vi "AlliGator Square Gated IRF Characteristics Map.vi"(8 "error in (no error)":errorcluster, 11 "AlliGator Internal Variables DVR":refnum<data-value>) -> (0 "error out":errorcluster, 1 "Message":string, 3 "AlliGator Internal Variables DVR":refnum<data-value>)   [LabVIEW 2021, in "AlliGator Scripts.lvlib"]
doc: "Performs a crude square gate analysis of all ROI decays and saves the gate parameters in an ASCII file."
uses:
  AlliGator Scripts.lvlib
  Internal Variables/AlliGator Internal Variables v2.ctl
  <vilib>/vision/Image Controls.llb/IMAQ Image.ctl
  Internal Variables/AlliGator Gate Image Set.ctl
  Files/AlliGator FLI Dataset Type.ctl
  Files/AlliGator Data Series Type.ctl
  Dual-Channel Datasets/AlliGator Dataset Channel.ctl
  Settings/AlliGator Gate Arithmetic.ctl
  Source Image/AlliGator Displayed Image.ctl
  Image/Named ROI Description.ctl
  Phasor Graph/AlliGator Decay Metadata v3.ctl
  Decay Analysis/Decay Preprocessing/AlliGator Decay Background Subtraction Info.ctl
  Decay Analysis/Decay Preprocessing/AlliGator Baseline Subtraction Method.ctl
  Graphs/XY Graph/XY Graph Plot Shift Parameters.ctl
  Graphs/XY Graph/XY Graph Plot Shift Method.ctl
  Decay Analysis/Decay Preprocessing/AlliGator Decay Extrapolation Parameters.ctl
  Phasor/Calibration Phasor (m, phi).ctl
  Phasor/Phasor Reference Series.ctl
  Phasor/Phasor Calibration Map v2.ctl
  Phasor/Phasor (g, s).ctl
  Phasor Graph/AlliGator Raw Phasor Plot Data v5.ctl
  Phasor/Phasor Standard Deviation Options.ctl
  Phasor Plot/AlliGator Phasor Multi-Harmonic Data.ctl
  Phasor/Phasor Harmonic Data.ctl
  Decay Fit Parameter Map/AlliGator Decay Fit Options & Parameters v4.ctl
  Fits/IRF(X)PSED/Decay Fit Options v4.ctl
  Fits/Decay Convolution/Decay Model.ctl
  Fits/Residual Type.ctl
  Fits/IRF(X)PSED/Fit Weights Type v2.ctl
  Fits/Non-linear Fitting Method v2.ctl
  Fits/Fit Calculation Method.ctl
  Fits/Non-linear Fitting Algorithm.ctl
  Decay Analysis/Decay Fit/AlliGator Decay Fit Parameter Constraints 2.ctl
  Fits/IRF(X)PSED/Decay Fit Parameters In List.ctl
  Fits/IRF(X)PSED/MLE Baseline Offset Type.ctl
  Decay Analysis/Decay Preprocessing/AlliGator Decay Preprocessing Parameters.ctl
  Fits/IRF(X)PSED/Decay Fit Parameters & Derived Quantities List v2.ctl
  Fits/IRF(X)PSED/Decay Fit Result Constraint.ctl
  Decay Fit Parameter Map/AlliGator Parameter Maps Data.ctl
  Globals, Variables, Constants/AlliGator Variables List.ctl
  Settings/AlliGator Settings List.ctl
  Fits/Square Pulse/Square Pulse Options.ctl
  Fits/Square Pulse/Square Pulse Levels Type.ctl
  Variant/Variant to Data/Variant to U16.vi
  Globals, Variables, Constants/AlliGator Abort.vi
  <vilib>/Utility/file.llb/Write Delimited Spreadsheet (string).vi
  <vilib>/Utility/error.llb/Error Cluster From Error Code.vi
  <vilib>/ErrorRing/Error Ring.xnode
  Globals, Variables, Constants/AlliGator Globals, Variables & Constants.lvlib
  Image/Image.lvlib
  Decay Analysis/Decay Processing/AlliGator Decay Processing.lvlib
  Source Image/AlliGator Source Image.lvlib
  Strings/Strings.lvlib
  Time/Time.lvlib
  Decay Analysis/Decay Preprocessing/AlliGator Decay Preprocessing.lvlib
  Settings/AlliGator Settings.lvlib
  Fits/Fits.lvlib
  GUI/GUI.lvlib
  Utilities/Utilities.lvlib
  Variant/Variant to Data/Variant to Data.lvlib
  Phasor/Phasor.lvlib
  Files/AlliGator Files.lvlib
  Internal Variables/AlliGator Internal Variables.lvlib
  Phasor Graph/AlliGator Phasor Graph.lvlib
  Graphs/XY Graph/XY Graph Add-Ons.lvlib
  Phasor Plot/AlliGator Phasor Plot.lvlib
  Decay Analysis/Decay Fit/AlliGator Decay Fit.lvlib
  Dual-Channel Datasets/AlliGator Dual-Channel Datasets.lvlib
  Decay Fit Parameter Map/AlliGator Decay Fit Parameter Map.lvlib
panel:
  # "see the AlliGator License on the block diagram (Ctrl+E or Window:Show Block Diagram)"
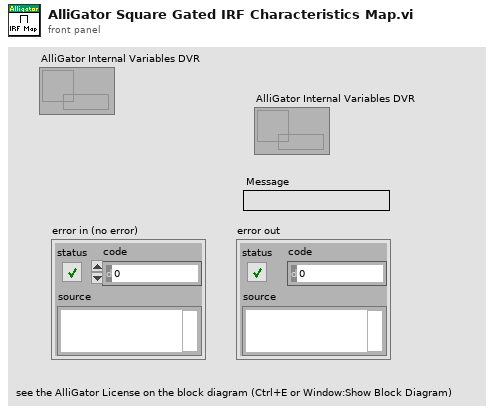
[diagram p1: front panel]
types:
  T1 = typedef "AlliGator Globals, Variables & Constants.lvlib/AlliGator Variables List.ctl" = enum16{"---- GUI ----", "GUI:Initialization Status", "GUI:State Indicators Refnum", "GUI:Original AlliGator Menu Items", "GUI:Current Action Loop State", "GUI:Script in progress", "GUI:Playback", "GUI:Loop Playback", "GUI:Search ROI Used", "GUI:Search ROI", "Decay Graph Max Legend Size", "Intensity Graph Max Legend Size", "Decay Statistics Graph Max Legend Size", "Phasor Graph Max Legend Size", "Phasor Ratio Graph Max Legend Size", "Lifetime Graph Max Legend Size", "---- Files ----", "Files:Export Dataset Frames as Individual Files", "Files:Show Batch Export Help Balloons", "Files:Frames in Dataset", "Files:ptu File Frame Start Indices", "Files:Current Frame in Dataset", "Files:Current Frame Timestamp", "Files:Dataset Loaded", "Files:Dataset Metadata", "Files:Dataset Channel", "Files:Dataset Data Description", "Files:Background Dataset Metadata", "Files:Background Dataset Channel", "Files:Background Dataset Data Description", "Files:Background File Subtraction", "Files:Background File Path", "Files:Background File Pile-up Correction", "Files:Background File Pixel Well Capacity", "Files:Background File Scaling Factor", "Files:Current Dataset Load Settings", "Files:Dataset Path", "Files:ICCD-specific Information", "Files:Macrotime Gate Separation", "------ Python Plugins ------", "Python Plugins:Information", "Python Plugins:Python Session", "Python Plugins:Valid Python Session?", "---- Source Image ----", "Source Image:ROIs", "Source Image:Current ROI", "Source Image:ROI Event Refnum", "X_Source Image:Display Range", "X_Source Image:Palette Information", "X_Source Image:Type of Displayed Image", "X_Time Gate Slider", "Source Image:Palette List", "Source Image:Scale", "Source Image:ROI Overlay Color", "Source Image:Overlay to Erase", "Source Image:Is Displayed Image Accumulated", "Source Image:White Light Image Modified", "Source Image:Mask Image Modified", "---- Image Profile Window ----", "Image Profile:Window Event Refnum", "Image Profile:IntensityType", "Image Profile:Intensity Average Type", "Image Profile:Intensity-weighted SDV", "Image Profile:Box Profile Type", "Image Profile:Window Open", "Image Profile:Plotted Fit Parameter", "------ Phasor Graph -------", "Phasor Graph:Show Line", "---- Phasor Plot ---", "Phasor Plot:Parameters Changed", "Phasor Plot:FLI Dataset Modified since last Calculation", "Phasor Harmonics Data", "Selected Phasor Harmonics", "Phasor Harmonic Manager Event Refnum", "Phasor Plot:ROIs", "Phasor Plot:Current ROI", "Phasor Plot:ROI Event Refnum", "Phasor Plot:Image Reference Points", "Phasor Plot:Computed", "Phasor Plot:Palette Information", "Phasor Plot:Palette List", "Phasor Plot:Phasor Ratio Palette Information", "Phasor Plot:Phasor Ratio Palette List", "Phasor Plot:Image Scale", "Phasor Plot:Image Overlay to Erase", "Phasor Plot:Image Elements to Update", "Phasor Plot:Current Calculation Parameters", "Phasor Plot:Current Calibration Options", "Phasor Plot:Reset Cumulated Phasor Plot", "Phasor Plot:Reference 1", "Phasor Plot:Lifetime Reference 1", "Phasor Plot:Reference 1 Frequency", "Phasor Plot:Reference 2", "Phasor Plot:Lifetime Reference 2", "Phasor Plot:Reference 2 Frequency", "---- Decay Analysis ----", "Number of Selected Decays to Fit", "LS Fit Results", "LAR Fit Results", "BS Fit Results", "Last Decay Max - Min", "Best Fit Parameters", "Best Fit Parameter Names", "Actual Size X", "Actual Size Y", "Binning X", "Binning Y", "Actual # Gates", "Dataset Number", "Gates to...", "Gates Skipped", "Gates to keep", "Gate Step", "Gate Separation", "Reversed Gates", "Pile-up Correction", "Pixel Well Capacity", "Background Subtracted", "Background Subtraction Method", "Background Definition Range", "Background File (deprecated)", "Number of Dataset Accumulated", "Array of Accumulated Dataset Paths", "Do Averaged Datasets", "Destination File Path", "Process Plot Target", "Use 1/D as Phasor Frequency", "---- Decay Fit Parameter Map -----", "Decay Fit Parameter Map:Palette Information", "Decay Fit Parameter Map:Palette List", "Decay Fit Parameter Map:X Resolution", "Decay Fit Parameter Map:Y Resolution", "Decay Fit Parameter Map:Use Decay Fit Result Constraints", "Decay Fit Parameter Map:Decay Fit Result Constraints", "Decay Fit Parameter Map:Decay Fit Result Constraints Applied", "---- Parameter Map ----", "Parameter Map:Palette Information", "Parameter Map:Palette List", "------- Local Decay Window ---------", "Local Decay Graph Window:Event Refnum", "Local Decay Graph Window:Use normalized IRF for convolution", "----- Miscellaneous ----", "Misc:Skippable Dialog Windows Status"}
  T2 = typedef "IMAQ Image.ctl" = refnum<image>
  T3 = typedef "AlliGator Settings.lvlib/AlliGator Settings List.ctl" = enum16{"GUI:Visible Settings Tab", "GUI:Last Run Version", "Source Image:Use Image Histogram for Contrast", "Source Image:Low Count Pixels Rejection Options", "Source Image:High Count Pixels Rejection Options", "Source Image:Use Image Brightness", "Source Image:Blend Overlay with Image Background", "Source Image:Use Fixed ROI Diameter", "Source Image:ROI Diameter", "Source Image:ROI Center Color", "Source Image:Peak Threshold", "Source Image:Intensity Threshold", "Source Image:Image Binning Options", "Source Image:Image Smoothing Options", "Source Image:Image Histogram Active", "Source Image:Invert Binary Mask", "Source Image:Hot Pixel Removal", "Source Image:Overlay Analyzed ROI Center", "Source Image:Auto-Adjust Contrast", "Source Image:Histogram Lower Percentile", "Source Image:Histogram Upper Percentile", "Source Image:Save Source Image", "Source Image:Scale Bar Options", "Source Image:Image Resolution (Pixel Size)", "Source Image:Flatfield Correction", "Source Image:Show Dead Left Columns Correction", "Source Image:Dead Left Columns Correction", "Source Image:Image Pre-Processing Operations Order", "Source Image:Overlay ROI Median", "Source Image:Median Overlay Color", "Data Information:Gate Width", "Data Information:Nanotime Gate Separation", "Data Information:Macrotime Gate Separation", "Data Information:Gate Step", "Data Information:# Gates", "Data Information:Gate Image Exposure", "Data Information:Gate Image Integration", "Data Information:Gates to Skip", "Data Information:Gates to Keep", "Data Information:Define Gates to", "Data Information:Channel Name", "Data Information:Available Channel Names", "Data Information:Channel Arithmetic", "Data Information:Background File Subtraction", "Data Information:Background File", "Data Information:Background Scaling Factor", "Data Information:Background Pile-up Correction", "Data Information:Background Pixel Well Capacity", "Data Information:Laser Period", "Data Information:SYNC Period", "Data Information:Pile-up Correction", "Data Information:Pixel Well Capacity", "Data Information:Dataset Scaling Factor", "Fluorescence Decay_Decay Pre-Processing:Reverse Gates", "Fluorescence Decay_Decay Pre-Processing:Verbose Decay Pre-Processing", "Fluorescence Decay_Decay Pre-Processing:Use Decay Pre-Processing", "Fluorescence Decay_Decay Pre-Processing:Background Subtraction", "Fluorescence Decay_Decay Pre-Processing:Background Definition Range", "Fluorescence Decay_Decay Pre-Processing:Baseline Subtraction Method", "Fluorescence Decay_Decay Pre-Processing:Decay Pre-Processing Operations Order", "Fluorescence Decay_Decay Pre-Processing:Smoothing Parameter", "Fluorescence Decay_Decay Pre-Processing:Shift Decay", "Fluorescence Decay_Decay Pre-Processing:Decay Shift Parameters", "Fluorescence Decay_Decay Pre-Processing:Fold Decay", "Fluorescence Decay_Decay Pre-Processing:# Folds", "Fluorescence Decay_Decay Pre-Processing:1-Normalize Decay", "Fluorescence Decay_Decay Pre-Processing:[0-1]-Normalize Decay", "Fluorescence Decay_Decay Pre-Processing:Smoothen Decay", "Fluorescence Decay_Decay Pre-Processing:Extrapolate Decay", "Fluorescence Decay_Decay Pre-Processing:Use Periodicity", "Fluorescence Decay_Decay Pre-Processing:Use Cursors", "Fluorescence Decay_Decay Pre-Processing:Tail Fraction", "Fluorescence Decay_Decay Pre-Processing:Head Fraction", "Fluorescence Decay_Decay Pre-Processing:Additional Points", "Fluorescence Decay_Decay Pre-Processing:Straighten Decay", "Fluorescence Decay_Decay Pre-Processing:Constant Background", "Fluorescence Decay_Decay Pre-Processing:Pixel-Normalize Decay", "Fluorescence Decay_Advanced Analysis:Extract IRF instead of Decay", "Fluorescence Decay_Advanced Analysis:IRF Extraction Options", "Fluorescence Decay_Advanced Analysis:IRF Optimization Options", "Fluorescence Decay_Advanced Analysis:Square Pulse Options", "Fluorescence Decay_Advanced Analysis:IRF Order", "Fluorescence Decay_Advanced Analysis:IRF Time Constants", "Fluorescence Decay_Advanced Analysis:Wavelet Analysis Options", "Fluorescence Decay_Advanced Analysis:Average Lifetime Options", "Fluorescence Decay_Fit Options:Fit Options", "Fluorescence Decay_Fit Options:Use Legacy Fitting Approach", "Fluorescence Decay_Fit Options:Use Data Information Laser Period", "Fluorescence Decay_Fit Parameters:Displayed Fit Parameters", "Fluorescence Decay_Fit Parameters:Fit Parameter Constraints", "Fluorescence Decay_Fit Parameters:Export Tabulated Results", "Fluorescence Decay_Fit Parameters:MLE Baseline Offset Type", "Fluorescence Decay_Fit Parameters:MLE Baseline Offset", "Fluorescence Decay_Fit Parameters:Guess Parameter Names", "Fluorescence Decay_Fit Parameters:Guess Parameter Values", "Fluorescence Decay_Fit Parameters:Guess Parameters Options", "Fluorescence Decay_Fit Parameters:Optimal Offset Selection Criterion", "Fluorescence Decay_Styles:Show Last Decay Only", "Fluorescence Decay_Styles:Decay Graph Color Array", "Fluorescence Decay:Decay Graph Active", "Fluorescence Decay Statistics:Min Peak Value", "Fluorescence Decay Statistics:Reject Low Decay Peak Pixels", "Fluorescence Decay Statistics:Reject High Decay Peak Pixels", "Fluorescence Decay Statistics:Max Peak Value", "Time Traces:Use File Timestamp", "Time Traces:Time Step", "Time Traces:Use Intensity Correction File", "Time Traces:Intensity Correction File", "Phasor Plot:Phasor Plot Smoothing Options", "Phasor Plot:Phasor Plot Size", "Phasor Plot:Phasor Plot Graphics Options", "Phasor Plot:Cumulative Phasor Plot", "Phasor Plot:Use Phasor Brightness", "Phasor Plot:Blend Overlay with Phasor Background", "Phasor Plot:Save Phasor Plot", "Phasor Plot:Show References", "Phasor Plot:Phasor Ratio Decay Range", "Phasor Plot:Exponential Fading", "Phasor Plot:Phasor Ratio Reference Colors", "Phasor Plot:Reference Radius", "Phasor Plot:Show Color Map Vertices", "Phasor Plot:Phasor Plot Active", "Phasor Plot:Phasor Ratio Color Map Type", "Phasor Plot:Phasor Ratio Color Map", "Phasor Plot:Phasor Ratio Display Range", "Phasor Plot:Selected Image ROI(s)", "Phasor Plot:All Image ROIs", "Phasor Plot:Selected Phasor Plot ROI(s)", "Phasor Plot:All Phasor Plot ROIs", "Phasor Plot:Phasor Ratio Color-Coded Quantity", "Phasor Plot:Store Phasor Harmonics", "Phasor Plot:Draw Reference Segment", "Phasor Plot:User-Defined Quantity", "Phasor Plot:Color Scale High Color", "Phasor Plot:Color Scale Low Color", "Phasor Plot:Intensity-weighted Phasor Plot", "Phasor Graph:Phasor Frequency", "Phasor Graph:Phasor Ratio Type", "Phasor Graph:Pixel-level Phasor Computation", "Phasor Graph:Save Phasor Graph", "Phasor Graph:Phasor Graph Active", "Phasor Graph:Phasor SDV Options", "Phasor Graph:Intensity-weighted Phasor Graph", "Phasor Graph:Define Shortest Lifetime as", "Phasor Calibration:Use Backup Calibration if needed", "Phasor Calibration:Backup Calibration Type", "Phasor Calibration:Calibration Type", "Phasor Calibration:Calibration Lifetime", "Phasor Calibration:Calibration Map Algorithm", "Single-Exponential Phasor Locus (SEPL):Gate Parameters", "Single-Exponential Phasor Locus (SEPL):User-defined Gate", "Single-Exponential Phasor Locus (SEPL):User-defined IRF", "Single-Exponential Phasor Locus (SEPL):Phasor Parameters", "Single-Exponential Phasor Locus (SEPL):Decay & IRF Parameters", "Single-Exponential Phasor Locus (SEPL):Display Parameters", "Lifetime Analysis:Decay Analysis Parameters", "Lifetime Analysis:Lifetime Map Active", "Plugins:Python Settings", "Miscellaneous:Verbose Mode", "Miscellaneous:Beep after Script", "Miscellaneous:Saved Image File Format", "Miscellaneous:Exported Gate Image Settings", "Miscellaneous:Include Loading in Timing", "Miscellaneous:Verbose Settings Mode", "Miscellaneous:Histogram Options", "Miscellaneous:Beep on Error", "Miscellaneous:# Logical Processors Used", "Miscellaneous:ROI Description Max Characters", "Miscellaneous:Verbose Error Mode", "Miscellaneous:Transparent Mask Color"}
  T4 = typedef "Fits.lvlib/Square Pulse Options.ctl" = cluster{"Method":T5, "# Bins":i32, "Threshold %":dbl, "Center on Midpoint":bool, "Smoothen Plot":bool}
  T5 = typedef "Fits.lvlib/Square Pulse Levels Type.ctl" = enum16{"Mode", "Mean"}
  T6 = typedef "Image.lvlib/Named ROI Description.ctl" = cluster{"ROI Descriptor":T7, "ROI Name":string, "Overlay Color":u32}
  T7 = typedef "ROI Descriptor" = cluster{"Global Rectangle":i32[], "Contours":cluster{"ID":enum32{"External", "Internal"}, "Type":u32, "Coordinates":i32[]}[]}
  T8 = typedef "AlliGator Internal Variables.lvlib/AlliGator Internal Variables v2.ctl" = cluster{"----------------------------- Images -----------------------------":u8, "Displayed Image":T2, "White Light Image":T2, "Mask Image":T2, "ROI Mask Image":T2, "Current Dataset Images 1":T9, "Background Dataset Images 1":T9, "Current Dataset Images 2":T9, "Background Dataset Images 2":T9, "Current Dataset Arithmetic Images":T9, "Accumulated Dataset Images 1":T9, "Accumulated Dataset Images 2":T9, "Accumulated Dataset Arithmetic Images":T9, "----------------------------- File Paths -----------------------------":u8, "Phasor Plot Image":T2, "Decay Fit Parameter Map Image":T2, "Parameter Map Image":T2, "Single Data Point Path":path, "White Light Image Path":path, "Mask Image Path":path, "Time-Series Folder":path, "[Time-Series Paths]":path[], "----------------------------- FLI Dataset -----------------------------":u8, "Current Dataset":i32, "Single Dataset Type":T10, "Current Folder":string, "AlliGator Data Series Type":T11, "# Datasets":i32, "Dual-Channel Dataset":bool, "Selected Channel Name":string, "Dataset Channel":T12, "Channel Arithmetic":T13, "Dual-Channel Background Dataset":bool, "Background Channel":T12, "Dual-Channel Accumulated Dataset":bool, "Start Time":dbl, "[Time-Series Timestamps]":dbl[], "[Intensity Corrections]":dbl[], "Time Series Script":bool, "Type of Displayed Image":T14, "Gate Image Slide":u16, "# Gates":i32, "ROIs":T6[], "----------------------------- Decays -----------------------------":u8, "ROI Decay":cluster{"t Array":dbl[], "I Array":dbl[]}, "Valid Decay":bool, "Decay  Metadata":T15, "Reference Decay Plot Name":string, "Reference Decay":cluster{"t Array":dbl[], "I Array":dbl[]}, "Decay Shift Plot":cluster{"Time Stamps":dbl[], "Decay Shifts":dbl[]}, "[Decays Max Values]":sgl[], "[Decays Min Values]":sgl[], "----------------------------- Calibration -----------------------------":u8, "Calibration Phasor":T21, "Calibration Phasor Series":T22, "Phasor Calibration Map":T23, "Calibration Map MD5 Digest":string, "----------------------------- Phasor Graph -----------------------------":u8, "Last Raw Phasor":T24, "Last Calibrated Phasor":T24, "Last Calibrated Phasor SDV":T24, "Phasor Graph:Phasor Plot":cluster{"g Array":dbl[], "s Array":dbl[]}, "Phasor Graph:Phasor SDV Plot":cluster{"g Array":dbl[], "s Array":dbl[]}, "[Phasor Graph:Raw Phasor Plots]":T25[], "Phasor Plot locked to Ref 1":i32, "[Phasor Plot(s) locked to Ref 1]":i32[], "[Phasor Plot(s) locked to Ref 2]":i32[], "[Pixel Phasors]":T24[], "----------------------------- Phasor Plot -----------------------------":u8, "[[Sum Image]]":dbl[][], "[[CSG Phasors]]":csg[][], "[[Valid Pixel?]]":bool[][], "[[Phasor Ratios]]":dbl[][], "[[Average Lifetimes]]":dbl[][], "Amplitude Weighted Average Lifetime":bool, "I/m/phi Dataset":cluster{"I/m/phi Dataset?":bool, "Base Frequency":dbl[unit], "Harmonic Orders":u8[]}, "Multi Phasor Plot Data":T27, "----------------------------- Decay Fit Parameter Map -----------------------------":u8, "Decay Fit Options & Parameters":T29, "Fit Options: Decay Preprocessing Parameters":T40, "Fit Options: Reference Decay":cluster{"t Array":dbl[], "I Array":dbl[]}, "Is Full Image Parameters Map":bool, "Is Single-Pixels Parameters Map":bool, "NLSF Parameters Map X Resolution":i32, "NLSF Parameters Map Y Resolution":i32, "[Single Decay Fit Parameters]":dbl[], "Fit Model":T31, "[[Multiple Decays Fit Parameters]]":dbl[][], "[[Multiple Decays Fit Parameter SDVs]]":dbl[][], "[[IRFs]]":dbl[][], "[ROI Descriptors]":T7[], "IRF Array Time Axis":dbl[], "Decay Array Time Axis":dbl[], "[Decay Fit Parameter Names]":T41[], "[Decay Sum]":dbl[], "Array of Decay Fit Result Constraints":T42[], "Selected ROIs Array":bool[], "----------------------------- Parameter Maps -----------------------------":u8, "[Map Set Names]":string[], "[Parameter Maps]":T43[], "[[User-defined Quantities]]":dbl[][], "User-defined Quantity":string}
  T9 = typedef "AlliGator Internal Variables.lvlib/AlliGator Gate Image Set.ctl" = cluster{"SGL Gate Images":T2[], "SGL Sum Image":T2, "SGL Max Image":T2, "SGL Min Image":T2}
  T10 = typedef "AlliGator Files.lvlib/AlliGator FLI Dataset Type.ctl" = enum16{"HDF5 FLI Dataset", "Gate Image Folder", ".sdt FLI Dataset (Becker & Hickl)", ".ptu FLI Dataset (PicoQuant)", "SS1 FLI Dataset", "SS2 FLI Dataset", "I/m/phi Dataset", ".bin FLI Dataset (PicoQuant Binned)", ".bin FLI Dataset (Piccolo Binned)", ".mat FLI Dataset"}
  T11 = typedef "AlliGator Files.lvlib/AlliGator Data Series Type.ctl" = enum16{"Not a Supported Series", "Gate Images Folder Series", "SwissSPAD 2 Dataset Series", "B&H FLI Dataset Series", "PicoQuant PTU FLI Dataset Series", "PicoQuant BIN FLI Dataset Series", "Piccolo hist BIN FLI Dataset Series", "HDF5 FLI Dataset Series"}
  T12 = typedef "AlliGator Dual-Channel Datasets.lvlib/AlliGator Dataset Channel.ctl" = enum16{"G2", "INT"}
  T13 = typedef "AlliGator Settings.lvlib/AlliGator Gate Arithmetic.ctl" = enum16{"None", "INT-G2", "G2/INT*<INT>", "(1 - G2/INT)*<INT>"}
  T14 = typedef "AlliGator Source Image.lvlib/AlliGator Displayed Image.ctl" = enum16{"Single Gate", "Sum of All Gates", "Max of All Gates", "Min of All Gates", "-", "White Ligth Image", "Mask Image"}
  T15 = typedef "AlliGator Phasor Graph.lvlib/AlliGator Decay Metadata v3.ctl" = cluster{"ROI Descriptor":T7, "ROI Center":cluster{"X":i32, "Y":i32}, "Decay Background Subtraction Info":T16, "Decay Reverted":bool, "Decay Smoothened":bool, "Decay Straightened":bool, "Fitted Tau (Decay Straightening)":dbl, "Decay Shift Parameters":T18, "Decay Shifted":bool, "Decay Extrapolated":bool, "Decay Extrapolation Parameters":T20, "Decay Normalized":bool, "Fold Decay":bool, "# Folds":u32}
  T16 = typedef "AlliGator Decay Preprocessing.lvlib/AlliGator Decay Background Subtraction Info.ctl" = cluster{"Laser Period":dbl[unit], "Gate Duration":dbl[unit], "Baseline Subtraction Method":T17, "Background Definition Range":cluster{"Min Gate":dbl[unit], "Max Gate":dbl[unit]}, "Total Intensity w/o Bkgd Subtraction":dbl, "Bkgd-subtracted Intensity (exp)":dbl, "# Data Points":i32, "Background/Gate":dbl, "Fitted Lifetime":dbl[unit], "Bkgd-subtracted Intensity (theo)":dbl}
  T17 = typedef "AlliGator Decay Preprocessing.lvlib/AlliGator Baseline Subtraction Method.ctl" = enum16{"Mean", "Min", "Square Gated Single-Exponential", "File", "Constant"}
  T18 = typedef "XY Graph Add-Ons.lvlib/XY Graph Plot Shift Parameters.ctl" = cluster{"Type":T19, "Shift":dbl[unit], "Threshold":dbl, "Rotate":bool}
  T19 = typedef "XY Graph Add-Ons.lvlib/XY Graph Plot Shift Method.ctl" = enum16{"Default", "CFD", "Threshold", "Cross-Correlation"}
  T20 = typedef "AlliGator Decay Preprocessing.lvlib/AlliGator Decay Extrapolation Parameters.ctl" = cluster{"Additional Points":u32, "Head Fraction":dbl, "Fitted Tau":dbl, "Use Periodicity":bool, "Use Cursors":bool, "Tail Fraction":dbl}
  T21 = typedef "Phasor.lvlib/Calibration Phasor (m, phi).ctl" = cluster{"m":dbl, "phi":dbl, "Phasor Frequency":dbl[unit], "Reference Lifetime":dbl[unit]}
  T22 = typedef "Phasor.lvlib/Phasor Reference Series.ctl" = cluster{"m Array":dbl[], "phi Array":dbl[], "Phasor Frequency":dbl[unit], "Calibration Lifetime":dbl[unit]}
  T23 = typedef "Phasor.lvlib/Phasor Calibration Map v2.ctl" = cluster{"Phasor Frequency":dbl[unit], "Calibration Lifetime":dbl[unit], "ROI Centers":cluster{"X":i32, "Y":i32}[], "ROI Descriptors":T7[], "Map Resolution X":i32, "Map Resolution Y":i32, "z Array":cdb[]}
  T24 = typedef "Phasor.lvlib/Phasor (g, s).ctl" = cluster{"g":dbl, "s":dbl}
  T25 = typedef "AlliGator Phasor Graph.lvlib/AlliGator Raw Phasor Plot Data v5.ctl" = cluster{"Phasor Plot Name":string, "Raw Phasor Plot":T24[], "Phasor Frequency":dbl[unit], "[Decay Metadata]":T15[], "Raw Phasor Plot SDV":T24[], "Phasor SDV Options":T26, "[Calibration Phasor]":T21[], "Intensity Array":dbl[]}
  T26 = typedef "Phasor.lvlib/Phasor Standard Deviation Options.ctl" = cluster{"Compute Estimated SDV":bool, "# Replicas":u32, "Use Estimated Average Phasor":bool}
  T27 = typedef "AlliGator Phasor Plot.lvlib/AlliGator Phasor Multi-Harmonic Data.ctl" = cluster{"Base Frequency":dbl[unit], "# Harmonics":u8, "Harmonic Orders":u8[], "Phasor Plot Settings Checksum":u64, "Phasor Harmonic Data Array":T28[]}
  T28 = typedef "Phasor.lvlib/Phasor Harmonic Data.ctl" = cluster{"Phasor Harmonic Name":string, "Phasor Plot Settings Checksum":u64, "Phasor Frequency":dbl[unit], "Base Frequency":dbl[unit], "Harmonic Order":u8, "Phasor Plot Parameters":string, "Phasor Array [[CSG]]":csg[][], "Dataset File Path":path}
  T29 = typedef "AlliGator Decay Fit Parameter Map.lvlib/AlliGator Decay Fit Options & Parameters v4.ctl" = cluster{"SYNC Period":dbl[unit], "Fit Options":T30, "Fit Parameter Constraints":T37[], "MLE Baseline Offset":dbl, "MLE Baseline Offset Type":T39}
  T30 = typedef "Fits.lvlib/Decay Fit Options v4.ctl" = cluster{"Show Fit Residuals":bool, "Fit Model":T31, "Residual Type":T32, "Max Decay Percentile":dbl, "Min Decay Percentile":dbl, "Show Full Decay":bool, "Weights":T33, "Fitting Method":T34, "Compute Parameter Uncertainties":bool, "Periodic Boundaries":bool, "Model Calculation":T35, "Period":dbl[unit], "Termination Criteria":cluster{"Max Iterations":i32, "Max Function Calls":i32, "Max Time":dbl[unit], "Function Tolerance":dbl, "Parameter Tolerance":dbl, "Gradient Tolerance":dbl, "Min Lambda":dbl, "Max Lambda":dbl, "Initial Tick Count":u32}, "Offset Resolution":dbl[unit], "Use Local IRF":bool, "Fitting Algorithm":T36, "Show Confidence Interval ":bool, "Confidence Level":dbl}
  T31 = typedef "Fits.lvlib/Decay Model.ctl" = enum16{"1-Exponential", "2-Exponentials"}
  T32 = typedef "Fits.lvlib/Residual Type.ctl" = enum16{"Standard", "Normalized", "Reduced"}
  T33 = typedef "Fits.lvlib/Fit Weights Type v2.ctl" = enum16{"Unweighted", "1/Variance (Neyman)", "1/Variance (Pearson)", "Best of All"}
  T34 = typedef "Fits.lvlib/Non-linear Fitting Method v2.ctl" = enum16{"Least Square", "Least Absolute Residual", "Bisquare", "MLE", "-", "Best of All"}
  T35 = typedef "Fits.lvlib/Fit Calculation Method.ctl" = enum16{"Simulation", "Convolution", "Integration"}
  T36 = typedef "Fits.lvlib/Non-linear Fitting Algorithm.ctl" = enum16{"Levenberg-Marquardt", "Trust-Region Dogleg"}
  T37 = typedef "AlliGator Decay Fit.lvlib/AlliGator Decay Fit Parameter Constraints 2.ctl" = cluster{"Fit Parameter":T38, "Min Value":dbl, "Max Value":dbl, "Global":bool, "Used":bool}
  T38 = typedef "Fits.lvlib/Decay Fit Parameters In List.ctl" = enum16{"Offset", "Baseline", "A_1", "tau_1", "A_2", "tau_2"}
  T39 = typedef "Fits.lvlib/MLE Baseline Offset Type.ctl" = enum32{"Absolute", "Percentage"}
  T40 = typedef "AlliGator Decay Preprocessing.lvlib/AlliGator Decay Preprocessing Parameters.ctl" = cluster{"Background Subtraction":bool, "Straighten Decay":bool, "Reverse Gates":bool, "1-Normalized Decay":bool, "Smoothen Decay":bool, "Smoothing Parameter":dbl, "Shift Decay":bool, "Decay Shift Parameters":T18, "Extrapolate Decay":bool, "Additional Points":u32, "Head Fraction":dbl, "Pixel-Normalize Decay":bool, "Use Periodicity":bool, "Use Cursors":bool, "Tail Fraction":dbl, "Use Decay Pre-Processing":bool, "Fold Decay":bool, "# Folds":u32, "[0-1]-Normalized Decay":bool}
  T41 = typedef "Fits.lvlib/Decay Fit Parameters & Derived Quantities List v2.ctl" = enum16{"Offset", "Baseline", "A_1", "tau_1", "A_2", "tau_2", "<tau>_a", "f1_a", "f2_a", "<tau>_i", "f1_i", "f2_i", "-", "R^2", "Chi^2"}
  T42 = typedef "Fits.lvlib/Decay Fit Result Constraint.ctl" = cluster{"Fit Parameter":enum16{"Offset", "Baseline", "A_1", "tau_1", "A_2", "tau_2", "<tau>_a", "f1_a", "f2_a", "<tau>_i", "f1_i", "f2_i", "-", "R^2", "Chi^2", "Max Relative Residual", "<Residual ACF>", "Residual ACF SDV", "tau_2/tau_1"}, "Min Value":dbl, "Max Value":dbl, "Use Constraint":bool}
  T43 = typedef "AlliGator Decay Fit Parameter Map.lvlib/AlliGator Parameter Maps Data.ctl" = cluster{"Map Set Name":string, "[Parameter Names]":string[], "[[Parameters]]":dbl[][], "[[Parameter SDVs]]":dbl[][], "Decay Array Time Axis":dbl[], "[[IRFs]]":dbl[][], "IRF Array Time Axis":dbl[], "X Resolution":i32, "Y Resolution":i32, "Intensity Array":dbl[]}
  T44 = typedef "AlliGator Settings.lvlib/AlliGator Pixel Counts Constraints.ctl" = cluster{"High Count Pixels Rejection Options":T45, "Low Count Pixels Rejection Options":T46}
  T45 = typedef "AlliGator Settings.lvlib/AlliGator High Count Pixels Rejection Options.ctl" = cluster{"Background High Threshold Factor":dbl, "Fixed High Background Threshold":dbl, "Reject High Count Pixels":bool, "High Percentile":dbl}
  T46 = typedef "AlliGator Settings.lvlib/AlliGator Low Count Pixels Rejection Options.ctl" = cluster{"Background Low Threshold Factor":dbl, "Fixed Low Background Threshold":dbl, "Reject Low Count Pixels":bool, "Low Percentile":dbl}
  T47 = cluster{"Decay Peak Constraint":bool, "Min":dbl, "Max":dbl}
  T48 = cluster{"t Axis":dbl[], "ROI Intensity Array":dbl[]}
  T49 = typedef "Fits.lvlib/Square Pulse Statistics.ctl" = cluster{"High Level":dbl, "Low Level":dbl, "Rising Edge Midpoint":dbl, "Falling Edge Midpoint":dbl, "Rising Edge Width":dbl, "Falling Edge Width":dbl}
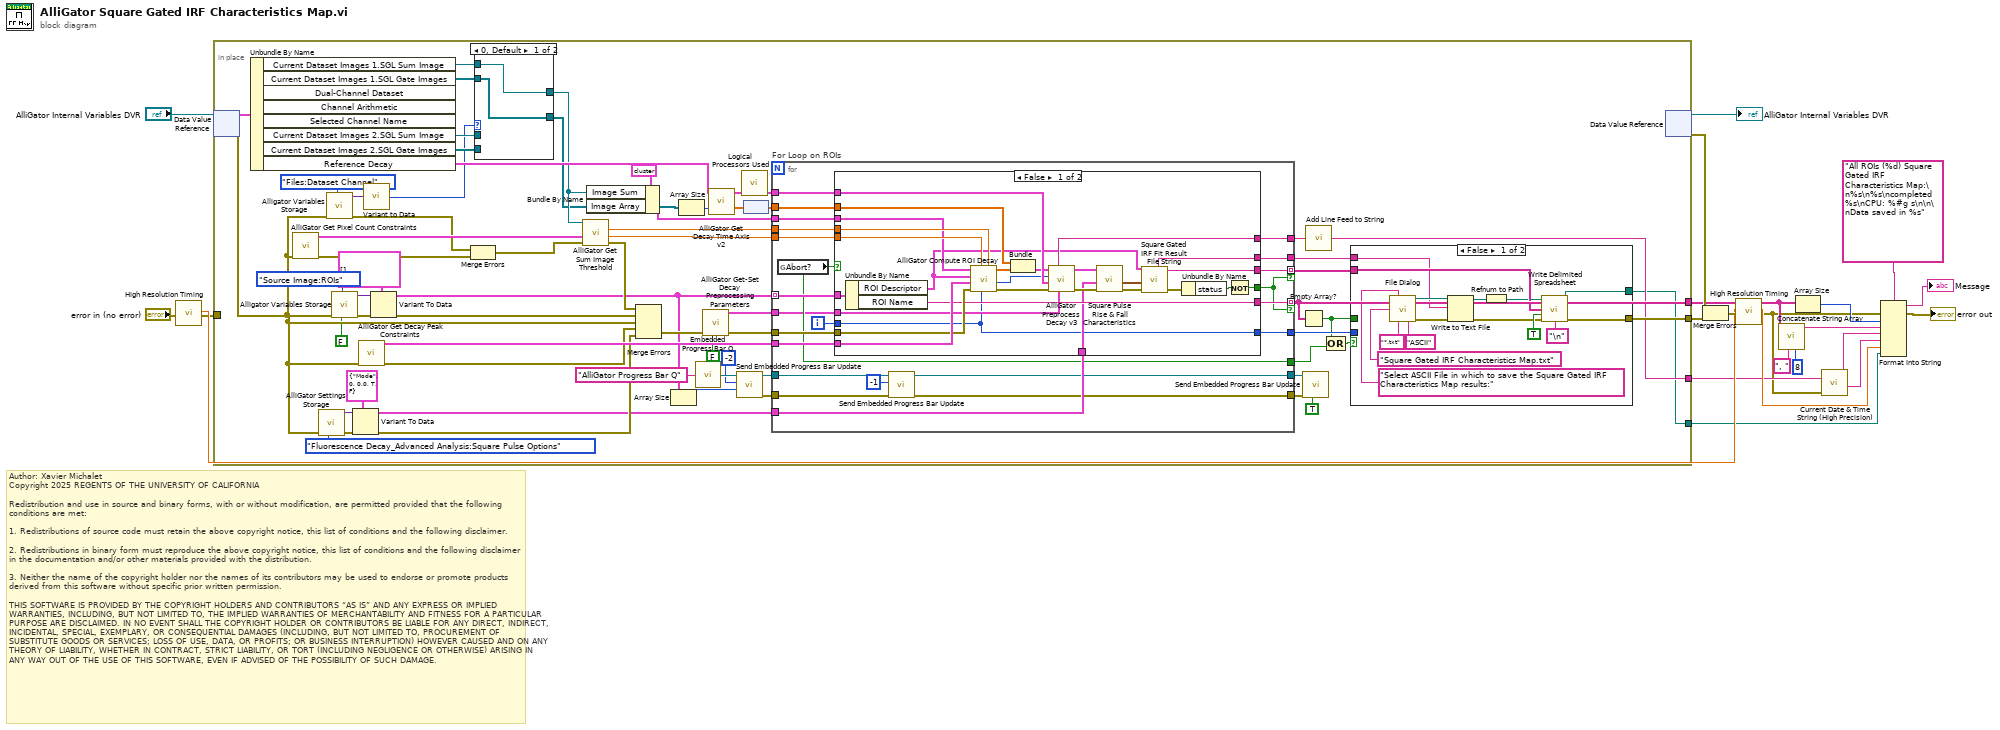
[diagram p0: block diagram]
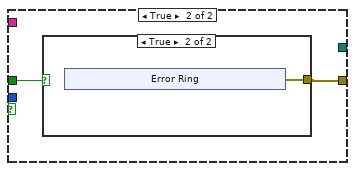
[diagram p2: hidden frame]
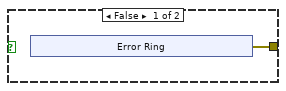
[diagram p3: hidden frame]
diagram:
  # "Author: Xavier Michalet\nCopyright 2025 REGENTS OF THE UNIVERSITY OF CALIFORNIA\n\nRedistribution and use in source and binary forms, with or without modification, are permitted provided that the following conditions are met:\n\n1. Redistributions of source code must retain the above copyright notice, this list of conditions and the following disclaimer.\n\n2. Redistributions in binary form must reproduce the above copyright notice, this list of conditions and the following disclaimer in the documentation and/or other materials provided with the distribution.\n\n3. Neither the name of the copyright holder nor the names of its contributors may be used to endorse or promote products derived from this software without specific prior written permission.\n\nTHIS SOFTWARE IS PROVIDED BY THE COPYRIGHT HOLDERS AND CONTRIBUTORS “AS IS” AND ANY EXPRESS OR IMPLIED WARRANTIES, INCLUDING, BUT NOT LIMITED TO, THE IMPLIED WARRANTIES OF MERCHANTABILITY AND FITNESS FOR A PARTICULAR PURPOSE ARE DISCLAIMED. IN NO EVENT SHALL THE COPYRIGHT HOLDER OR CONTRIBUTORS BE LIABLE FOR ANY DIRECT, INDIRECT, INCIDENTAL, SPECIAL, EXEMPLARY, OR CONSEQUENTIAL DAMAGES (INCLUDING, BUT NOT LIMITED TO, PROCUREMENT OF SUBSTITUTE GOODS OR SERVICES; LOSS OF USE, DATA, OR PROFITS; OR BUSINESS INTERRUPTION) HOWEVER CAUSED AND ON ANY THEORY OF LIABILITY, WHETHER IN CONTRACT, STRICT LIABILITY, OR TORT (INCLUDING NEGLIGENCE OR OTHERWISE) ARISING IN ANY WAY OUT OF THE USE OF THIS SOFTWARE, EVEN IF ADVISED OF THE POSSIBILITY OF SUCH DAMAGE."
  n1 = call "High Resolution Timing.vi"("Error In"="error in (no error)") -> ("elapsed (relative) seconds"=w12:dbl, "Error Out"=w7:errorcluster)  [unwired: 16 in, 1 out]
  n2 = in-place {
    in-place-border: [w83] -> w17
    in-place-border: [w82] -> w9
    in-place-border: w7 -> [_]
    in-place-border: [w80] -> w6
    in-place-border: [w79] -> w4
    n3 = in-place-dvr #1("AlliGator Internal Variables DVR") -> (w84:T8, w81:errorcluster)
    n4 = Unbundle By Name(w84) -> ("Current Dataset Images 1.SGL Sum Image"=w33:T2, "Current Dataset Images 1.SGL Gate Images"=w30:T2[], "Current Dataset Images 2.SGL Sum Image"=w28:T2, "Current Dataset Images 2.SGL Gate Images"=w31:T2[], "Reference Decay"=w63:cluster{"t Array":dbl[], "I Array":dbl[]})  [unwired: 3 out]
    n5 = call "AlliGator Get Pixel Count Constraints.vi"("error in (no error)"=w81) -> ("error out"=w72:errorcluster, "Pixel Count Constraints"=w73:T44)  [unwired: 9 in]
    n6 = call "AlliGator Settings Storage.vi"("AlliGator Settings List"=AlliGator_Settings_List."Fluorescence Decay_Advanced Analysis:Square Pulse Options", "Error In"=w81) -> ("Error Out"=w52:errorcluster, "Variant Data out"=w50:variant)  [unwired: 8 in]
    n7 = call "Alligator Variables Storage.vi"("AlliGator Variable"=AlliGator_Variables_List."Files:Dataset Channel" ("Alligator Variable"), "Error In"=w81) -> ("Error Out"=w23:errorcluster, "Data out"=w25:variant)  [unwired: 7 in, 1 out]
    n8 = call "Alligator Variables Storage.vi"("Get(F)/Set"=FALSE, "AlliGator Variable"=AlliGator_Variables_List."Source Image:ROIs" ("Alligator Variable"), "Error In"=w81) -> ("Error Out"=w76:errorcluster, "Data out"=w77:variant)  [unwired: 6 in, 1 out]
    n9 = Variant To Data(error in=w52, type=T4 {"Method"=enum."Mode", "# Bins"=0, "Threshold %"=0.0, "Center on Midpoint"=TRUE, "Smoothen Plot"=FALSE} ("Square Pulse Options"), Variant=w50) -> (data=w48:T4, error out=w49:errorcluster)
    n10 = call "AlliGator Get Decay Peak Constraints.vi"("error in (no error)"=w81) -> ("Error Out"=w56:errorcluster, "Decay Peak Constraints"=w68:T47)  [unwired: 9 in]
    n11 = call-poly "Variant to Data.vi"("Variant"=w25) -> ("U16 Value"=w22:u16)  [unwired: 8 in]
    n12 = Variant To Data(error in=w76, type=T6[] [] ("Stored ROIs in"), Variant=w77) -> (data=w38:T6[], error out=w71:errorcluster)
    n13 = Merge Errors(w23, w72) -> (w24:errorcluster)
    n14 = case shown="0, Default" w22 {
      tunnel: [w163 w165] -> w32
      tunnel: w28 -> [_ w165]
      tunnel: [w162 w164] -> w29
      tunnel: w31 -> [_ w164]
      tunnel: w33 -> [w163 _]
      tunnel: w30 -> [w162 _]
      frame 0, Default {
      }
      frame 1 {
      }
    }
    n15 = call "AlliGator Get Sum Image Threshold.vi"("error in (no error)"=w24, "Pixel Counts Constraints"=w73, "Image in"=w32) -> ("error out"=w58:errorcluster, "Pixel Threshold Low"=w69:sgl, "Pixel Threshold High"=w70:sgl)  [unwired: 2 in, 4 out]
    n16 = Bundle By Name(cluster=cluster{"Image Sum":T2, "Image Array":T2[]} {"Image Sum"=refnum, "Image Array"=[]} ("Images"), "Image Sum"=w32, "Image Array"=w29) -> (w67:cluster{"Image Sum":T2, "Image Array":T2[]})
    n17 = Merge Errors(w58, w71, w81, w56, w49) -> (w47:errorcluster)
    n18 = Array Size(array=w38) -> (size(s)=w37:i32)
    n19 = Array Size(array=w29) -> (size(s)=w65:i32)
    n20 = call "Embedded Progress Bar Q.vi"("Progress Bar Queue Name"="AlliGator Progress Bar Q") -> ("Progress Bar Queue"=w44:refnum<queue>)  [unwired: 6 in]
    n21 = call "AlliGator Get-Set Decay Preprocessing Parameters.vi"("Get (F)/Set"=FALSE, "Error In"=w47) -> ("Error Out"=w46:errorcluster, "Decay Preprocessing Parameters out"=w35:T40)  [unwired: 8 in]
    n22 = call "AlliGator Get Decay Time Axis v2.vi"("Number of Gates"=w65) -> ("t Array"=w64:dbl[unit][])  [unwired: 14 in]
    n23 = call "Send Embedded Progress Bar Update.vi"("Max Iterations N"=w37, "Current Iteration i (i or -1: standard or || iteration; 0 or -2: first standard or || iteration)"=-2 ("Current Iteration i (i or -1: standard or || iteration; 0 or -2: first standard or || iteration)"), "Progress Bar Queue in"=w44) -> ("Error Out"=w41:errorcluster, "Progress Bar Queue out"=w43:refnum<queue>)  [unwired: 7 in]
    n24 = call "Logical Processors Used.vi"() -> ()  [unwired: 6 in, 1 out]
    n25 = node(w64) -> (w57:dbl[])
    n26 = for "For Loop on ROIs" {
      tunnel: w38 -> [w134] mode=indexing
      tunnel: w70 -> [w133]
      tunnel: w69 -> [w132]
      tunnel: w67 -> [w131]
      tunnel: w68 -> [w130]
      tunnel: [w120] -> w62
      tunnel: w57 -> [w126]
      tunnel: w63 -> [w127]
      tunnel: [w112] -> w61
      tunnel: [w128] -> w82 mode=indexing if=w123
      tunnel: w46 -> [w129]
      tunnel: [w125] -> w59
      tunnel: [w124] -> w55 mode=indexing if=w123
      tunnel: [w122] -> w54
      tunnel: w48 -> [w121]
      tunnel: w43 -> [w119]
      tunnel: [w118] -> w42
      tunnel: w41 -> [w117]
      tunnel: [w116] -> w40
      tunnel: w35 -> [w114]
      i -> [w113]
      n27 = global read "AlliGator Abort.vi" "Abort?"() -> (w120:bool)
      n28 = case shown="False" w120 {
        tunnel: w134 -> [w161 _]
        tunnel: w133 -> [w160 _]
        tunnel: w132 -> [w159 _]
        tunnel: w131 -> [w158 _]
        tunnel: w130 -> [w157 _]
        tunnel: w129 -> [w156 _]
        tunnel: [w155 _] -> w128
        tunnel: w127 -> [w153 _]
        tunnel: w126 -> [w151 _]
        tunnel: [w148 _] -> w125
        tunnel: [w143 _] -> w124
        tunnel: [w142 _] -> w123
        tunnel: [w140 _] -> w122
        tunnel: w121 -> [w139 _]
        tunnel: w114 -> [w136 _]
        tunnel: w113 -> [w135 _]
        tunnel: [w135 _] -> w112
        frame False {
          n29 = Unbundle By Name(w161) -> ("ROI Descriptor"=w141:T7, "ROI Name"=w155:string)
          n30 = call "AlliGator Compute ROI Decay.vi"("Pixel Threshold High"=w160, "Loop ID"=w135, "Pixel Threshold Low"=w159, "error in (no error)"=w156, "Decay Peak  Constraints"=w157, "ROI Descriptor"=w141, "Images"=w158) -> ("error out"=w152:errorcluster, "# Valid Pixels"=w137:i32, "Decay Points"=w150:dbl[])  [unwired: 2 out]
          n31 = Bundle(w151, "Decay Points"=w150) -> (w149:cluster{dbl[], "Decay Points":dbl[]})  [unwired: 1 in]
          n32 = call "AlliGator Preprocess Decay v3.vi"("Decay Preprocessing Parameters"=w136, "Error In"=w152, "Time-Gated Reference Decay"=w153, "# Pixels"=w137, "Decay (in)"=w149) -> ("Error Out"=w147:errorcluster, "Decay (out)"=w146:T48, "Message"=w148:string)  [unwired: 3 in, 1 out]
          n33 = call "Square Pulse Rise & Fall Characteristics.vi"("error in (no error)"=w147, "Square Pulse Options"=w139, "Decay"=w146) -> ("error out"=w145:errorcluster, "Square Pulse Statistics"=w138:T49)  [unwired: 4 in, 3 out]
          n34 = call "Square Gated IRF Fit Result File String.vi"("error in (no error)"=w145, "Square Pulse Statistics"=w138, "ROI Descriptor"=w141) -> ("error out"=w144:errorcluster, "Result String"=w143:string, "Header String"=w140:string)  [unwired: 6 in]
          n35 = Unbundle By Name(w144) -> ("status"=w154:bool)
          n36 = Not(x=w154) -> (.not. x?=w142:bool)
        }
        frame True {
        }
      }
      n37 = call "Send Embedded Progress Bar Update.vi"("Error In"=w117, "Current Iteration i (i or -1: standard or || iteration; 0 or -2: first standard or || iteration)"=-1 ("Current Iteration i (i or -1: standard or || iteration; 0 or -2: first standard or || iteration)"), "Progress Bar Queue in"=w119) -> ("Error Out"=w116:errorcluster, "Progress Bar Queue out"=w118:refnum<queue>)  [unwired: 7 in]
    }
    n38 = Empty Array?(array=w82) -> (empty?=w27:bool)
    n39 = call "Send Embedded Progress Bar Update.vi"("Stop Progress Bar (F)"=TRUE, "Error In"=w40, "Progress Bar Queue in"=w42) -> ()  [unwired: 7 in, 2 out]
    n40 = call "Add Line Feed to String.vi"("String"=w59) -> ("String\\n"=w80:string)  [unwired: 8 in]
    n41 = Compound Arithmetic op=OR(w27, w62) -> (w60:bool)
    n42 = case shown="False" w60 {
      tunnel: [w89 w101] -> w83
      tunnel: w61 -> [_ _]
      tunnel: w55 -> [w92 _]
      tunnel: w54 -> [w86 _]
      tunnel: [w85 _] -> w79
      tunnel: w27 -> [_ w100]
      frame False {
        n43 = call "File Dialog"("prompt"="Select ASCII File in which to save the Square Gated IRF Characteristics Map results:" ("prompt (Choose or enter file path)"), "default name"="Square Gated IRF Characteristics Map.txt", "pattern (all files)"="*.txt", "pattern label"="ASCII") -> ("selected path"=w94:path, "error out"=w99:errorcluster)  [unwired: 8 in, 2 out]
        n44 = Write to Text File(file (use dialog)=w94, text=w86, error in=w99) -> (refnum out=w88:refnum<file>, error out=w90:errorcluster)  [unwired: 1 in, 1 out]
        n45 = Refnum to Path(1:w88) -> (0:w87:path)
        n46 = call-poly <vilib>:"Write Delimited Spreadsheet.vi"("file path (dialog if empty)"=w87, "1D data"=w92, "append to file? (new file:F)"=TRUE, "error in (no error)"=w90, "delimiter (\\t)"="\n" ("delimiter (\\t)")) -> ("new file path (Not A Path if cancelled)"=w85:path, "error out"=w89:errorcluster)  [unwired: 9 in]
      }
      frame True {
        n47 = case shown="True" w100 {
          tunnel: [w102 w107] -> w101
          frame False {
            n48 = xnode "Error Ring"() -> ("error out"=w102:errorcluster)
          }
          frame True {
            n49 = xnode "Error Ring"() -> ("error out"=w107:errorcluster)
          }
        }
      }
    }
    n50 = in-place-dvr #1() -> (→"AlliGator Internal Variables DVR":refnum<data-value>, w18:errorcluster)  [unwired: 1 in]
  }
  n51 = Merge Errors(w18, w17) -> (w14:errorcluster)
  n52 = call "High Resolution Timing.vi"("relative seconds (NaN)"=w12, "Error In"=w14) -> ("elapsed (relative) seconds"=w11:dbl, "Error Out"=w5:errorcluster)  [unwired: 15 in, 1 out]
  n53 = call "Concatenate String Array.vi"("Max Number of Elements (None: -1)"=8 ("Max Number of Elements (None: 1)"), "Separator (TAB)"=", ", "String Array"=w9) -> ("Formatted String"=w10:string)  [unwired: 8 in]
  n54 = Array Size(array=w9) -> (size(s)=w8:i32)
  n55 = call "Current Date & Time String (High Precision).vi"("Error In"=w5) -> ("on <Date> at <Time>"=w1:string)  [unwired: 7 in, 3 out]
  n56 = Format Into String(format string="All ROIs (%d) Square Gated IRF Characteristics Map:\n%s\n%s\ncompleted %s\nCPU: %#g s\n\n\nData saved in %s", error in=w5, w8, w10, w6, w1, w11, w4) -> (resulting string=→"Message":string, error out=→"error out":errorcluster)  [unwired: 1 in]
